vi "IfElse.vi"() -> ()   [LabVIEW 2020]
panel:
  out "GreaterThan10":bool
  out "LessThan10":bool
  in  "Dial":dbl(knob) scale=0.0..10.0
  in  "Slide":dbl(slide) scale=0.0..10.0
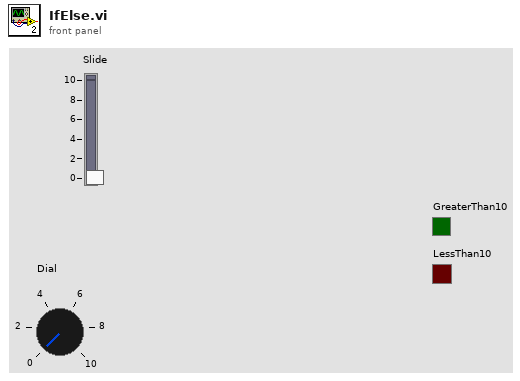
[diagram p1: front panel]
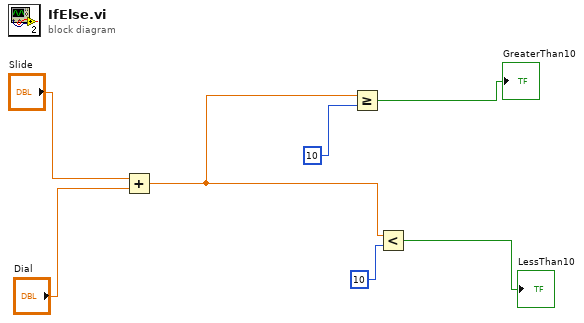
[diagram p0: block diagram]
diagram:
  n1 = Add(x="Slide", y="Dial") -> (x+y=w3:dbl)
  n2 = Greater Or Equal?(x=w3, y=10) -> (x >= y?=→"GreaterThan10":bool)
  n3 = Less?(x=w3, y=10) -> (x < y?=→"LessThan10":bool)
